vi "rcpacini_0_explore.vi"(6 "Variant in":variant, 7 "Shift Pressed?":bool, 8 "error in (no error)":errorcluster, 10 "QD Combo Box Ref":refnum<vi>, 11 "QD Launch VI Ref":refnum<vi>) -> (0 "error out":errorcluster, 4 "Variant out":variant)   [LabVIEW 2019]
doc: "Open in file explorer.\n\nCreated by: Ryan Pacini\n\nDefault Shortcut - [0]"
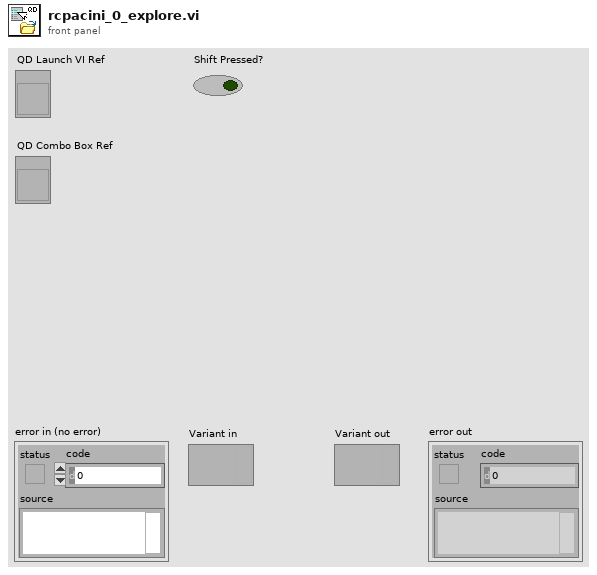
[diagram p1: front panel]
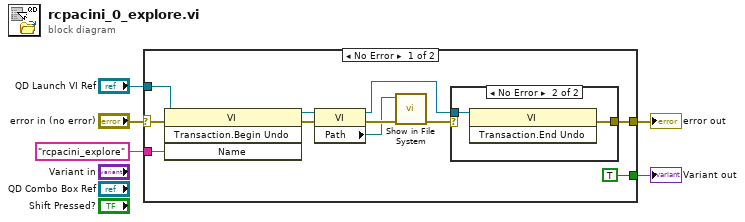
[diagram p0: block diagram]
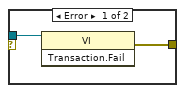
[diagram p2: hidden frame]
diagram:
  n1 = case shown="No Error" "error in (no error)" {
    selector: "error in (no error)" -> [w16 w21]
    tunnel: [w15 w21] -> w1
    tunnel: "QD Launch VI Ref" -> [w12 _]
    tunnel: "rcpacini_explore" ("Undo Name") -> [w14 _]
    tunnel: [TRUE _] -> w2
    frame No Error {
      n2 = invoke class="VI" method="Transaction.Begin Undo"(reference=w12, error in=w16, "Name"=w14) -> (reference out=w10:refnum<vi>, error out=w11:errorcluster)  [unwired: 1 in, 2 out]
      n3 = property class="VI"(reference=w10, error in=w11) -> (reference out=w6:refnum<vi>, error out=w9:errorcluster, "Path"=w8:path)
      n4 = call <vilib>:"Show in File System.vi"("error in (no error)"=w9, "file or directory path"=w8) -> ("error out"=w7:errorcluster)  [unwired: 9 in]
      n5 = case shown="No Error" w7 {
        tunnel: w6 -> [w17 w19]
        tunnel: [w18 w20] -> w15
        frame Error {
          n6 = invoke class="VI" method="Transaction.Fail"(reference=w17) -> (error out=w18:errorcluster)  [unwired: 2 in, 2 out]
        }
        frame No Error {
          n7 = invoke class="VI" method="Transaction.End Undo"(reference=w19) -> (error out=w20:errorcluster)  [unwired: 2 in, 2 out]
        }
      }
    }
    frame Error {
    }
  }
  "error out" <- w1
  "Variant out" <- w2
